vi "Register User Events.vi"(8 "error in (no error)":errorcluster, 11 "SongQueueActor in":refnum<class "SongQueueActor.lvclass">) -> (0 "error out":errorcluster, 3 "SongQueueActor out":refnum<class "SongQueueActor.lvclass">, 5 "Event Registration Refnum":refnum<event-registration>, 7 "Exit Event":refnum<user-event>)   [LabVIEW 2015, in "SongQueueActor.lvlib" / "SongQueueActor.lvclass"]
uses:
  SongQueueActor.lvclass
  SongQueueActor.lvclass/SongQueueActor.ctl
  builds/xctls/Song Queue/Song Queue.lvlibp/app/xctls/SongQueue/Song Queue.xctl
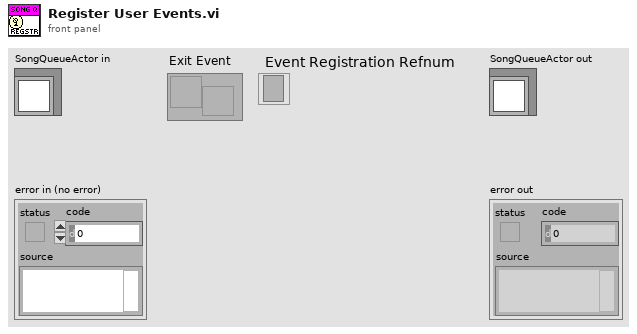
[diagram p1: front panel]
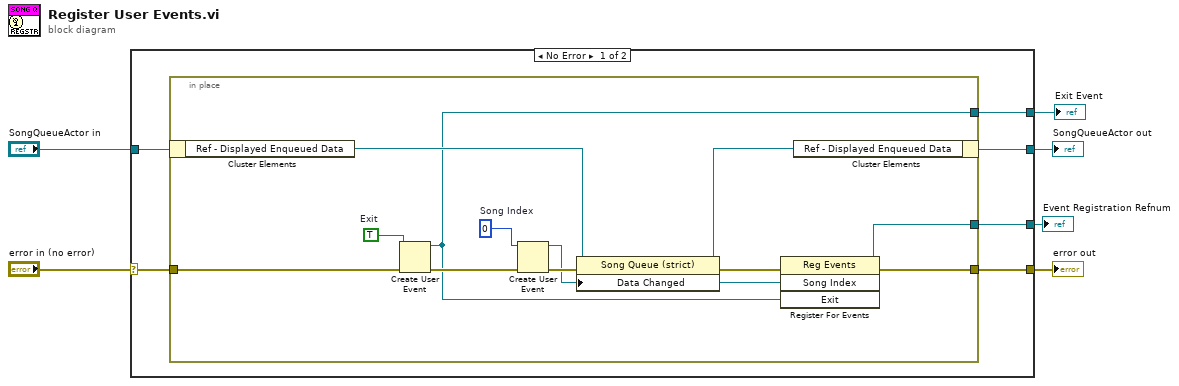
[diagram p0: block diagram]
diagram:
  n1 = case shown="No Error" "error in (no error)" {
    selector: "error in (no error)" -> [w10 w26]
    tunnel: [w12 w26] -> w5
    tunnel: [w9 w25] -> w3
    tunnel: "SongQueueActor in" -> [w11 w25]
    tunnel: [w8 _] -> w2
    tunnel: [w7 _] -> w1
    frame No Error {
      n2 = in-place {
        in-place-border: [w24] -> w12
        in-place-border: w10 -> [w19]
        in-place-border: [w16] -> w8
        in-place-border: [w15] -> w7
        w14 = u32 0  # Song Index
        w18 = TRUE  # Exit
        n3 = in-place-cluster #1(w11) -> ("Ref - Displayed Enqueued Data"=w22:refnum<vi>)
        n4 = Create User Event(user event datatype=w18, error in=w19) -> (user event=w16:refnum<user-event>, error out=w17:errorcluster)
        n5 = Create User Event(user event datatype=w14, error in=w17) -> (user event=w13:refnum<user-event>, error out=w20:errorcluster)
        n6 = property on="Property Node" class="Song Queue (strict)"(reference=w22, error in=w20, "Data Changed"=w13) -> (reference out=w21:refnum<vi>, error out=w23:errorcluster)
        n7 = register-events(error in=w23, w13, w16) -> (reference out=w15:refnum<event-registration>, error out=w24:errorcluster)  [unwired: 1 in]
        n8 = in-place-cluster #1("Ref - Displayed Enqueued Data"=w21) -> (w9:refnum<class "SongQueueActor.lvclass">)
      }
    }
    frame Error {
    }
  }
  "error out" <- w5
  "SongQueueActor out" <- w3
  "Exit Event" <- w2
  "Event Registration Refnum" <- w1
